vi "query setpoint.vi"(8 "error in (no error)":errorcluster, 11 "VISA session":refnum<visa-resource-name>) -> (0 "error out":errorcluster, 2 "Setpoint":dbl[unit], 3 "dup VISA session":refnum<visa-resource-name>)   [LabVIEW 2023]
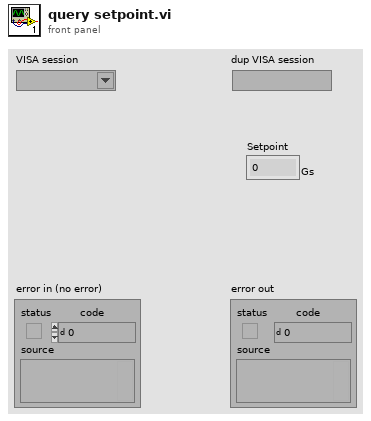
[diagram p1: front panel]
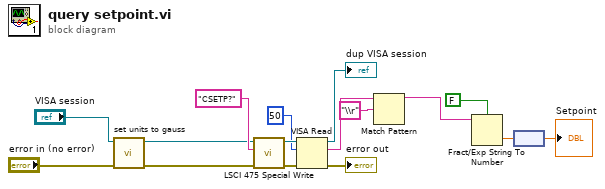
[diagram p0: block diagram]
diagram:
  n1 = call "set units to gauss.vi"("VISA session"="VISA session", "error in (no error)"="error in (no error)") -> ("dup VISA session"=w5:refnum<visa-resource-name>, "error out"=w3:errorcluster)  [unwired: 7 in]
  n2 = call "LSCI 475 Special Write.vi"("error in (no error)"=w3, "Write Buffer (\"\")"="CSETP?", "VISA session"=w5) -> ("error out"=w13:errorcluster, "dup VISA session"=w14:refnum<visa-resource-name>)  [unwired: 6 in, 1 out]
  n3 = VISA Read(VISA resource name=w14, byte count=u32 50, error in (no error)=w13) -> (VISA resource name out=→"dup VISA session":refnum<visa-resource-name>, read buffer=w11:string, error out=→"error out":errorcluster)  [unwired: 1 out]
  n4 = Match Pattern(string=w11, regular expression="\\r") -> (before substring=w7:string)  [unwired: 1 in, 3 out]
  n5 = Fract/Exp String To Number(use system decimal point (T)=FALSE, string=w7) -> (number=w1:dbl)  [unwired: 2 in, 1 out]
  n6 = node(w1) -> (→"Setpoint":dbl[unit])
